vi "SetItemColor.vi"(8 "エラー入力(エラーなし)":errorcluster, 9 "行列指定":T1={"Row"=-2, "Column"=-2}, 10 "色指定":cluster{"背景色":u32, "文字色":u32}={"背景色"=16448250, "文字色"=0}, 11 "Tbl refnum":refnum<vi>) -> (0 "エラー出力":errorcluster, 3 "Tbl refnum出力":refnum<vi>)   [LabVIEW 2014]
uses:
  <vilib>/Utility/miscctls.llb/LVRowAndColumnTypeDef.ctl
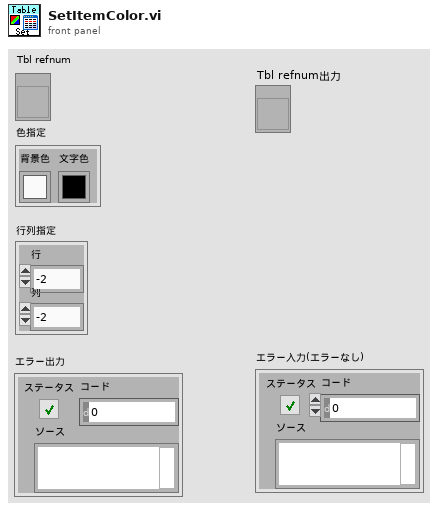
[diagram p1: front panel]
types:
  T1 = typedef "LVRowAndColumnTypeDef.ctl" = cluster{"Row":i32, "Column":i32}
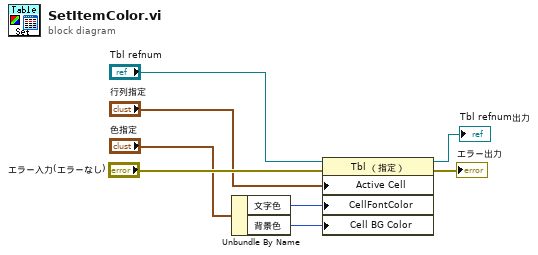
[diagram p0: block diagram]
diagram:
  n1 = Unbundle By Name("色指定") -> ("文字色"=w3:u32, "背景色"=w2:u32)
  n2 = property class="Tbl （指定）"(reference="Tbl refnum", error in="エラー入力(エラーなし)", "Active Cell"="行列指定", "CellFontColor"=w3, "Cell BG Color"=w2) -> (reference out=→"Tbl refnum出力":refnum<vi>, error out=→"エラー出力":errorcluster)
